vi "test_TCP_3_RT.vi"() -> ()   [LabVIEW 2014]
panel:
  out "error out":errorcluster
  in  "stop":bool
  out "string":string
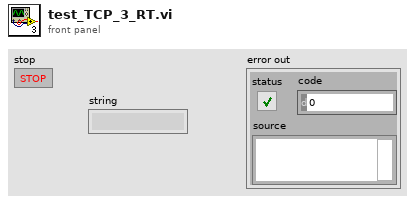
[diagram p1: front panel]
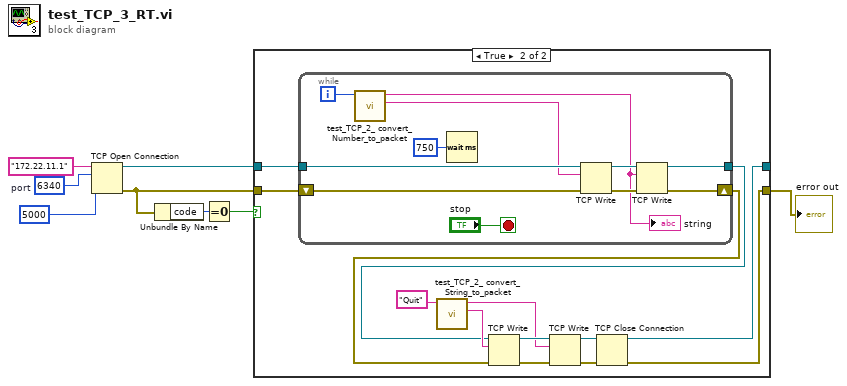
[diagram p0: block diagram]
diagram:
  w8 = u16 6340  # port
  n1 = TCP Open Connection(address="172.22.11.1", remote port or service name=w8, timeout ms (60000)=5000) -> (connection ID=w3:refnum<k5>, error out=w2:errorcluster)  [unwired: 2 in]
  n2 = Unbundle By Name(w2) -> ("code"=w5:i32)
  n3 = Equal To 0?(x=w5) -> (x = 0?=w4:bool)
  n4 = case shown="True" w4 {
    tunnel: w3 -> [w10 w23]
    tunnel: w2 -> [w9 w22]
    tunnel: [w10 w12] -> _
    tunnel: [w9 w11] -> w1
    frame False {
    }
    frame True {
      n5 = while {
        tunnel: w23 -> [w29]
        shift-right: [w33] -> w14
        shift-left: w22 -> [w30]
        tunnel: [w32] -> w13
        i -> [w26]
        stop <- "stop" stop-if-true
        n6 = call "test_TCP_2_ convert_Number_to_packet.vi"("input_Number"=w26) -> ("output_PrePacket"=w24:string, "output_packet"=w25:string)  [unwired: 9 in]
        "string" <- w25
        n7 = Wait (ms)(milliseconds to wait=u32 750) -> ()  [unwired: 1 out]
        n8 = TCP Write(connection ID=w29, data in=w24, error in (no error)=w30) -> (connection ID out=w27:refnum<k5>, error out=w28:errorcluster)  [unwired: 1 in, 1 out]
        n9 = TCP Write(connection ID=w27, data in=w25, error in (no error)=w28) -> (connection ID out=w32:refnum<k5>, error out=w33:errorcluster)  [unwired: 2 out]
      }
      n10 = call "test_TCP_2_ convert_String_to_packet.vi"("input_string"="Quit" ("data in")) -> ("output_PrePacket"=w21:string, "output_packet"=w18:string)  [unwired: 9 in]
      n11 = TCP Write(connection ID=w13, data in=w21, error in (no error)=w14) -> (connection ID out=w20:refnum<k5>, error out=w19:errorcluster)  [unwired: 2 out]
      n12 = TCP Write(connection ID=w20, data in=w18, error in (no error)=w19) -> (connection ID out=w16:refnum<k5>, error out=w15:errorcluster)  [unwired: 2 out]
      n13 = TCP Close Connection(connection ID=w16, error in (no error)=w15) -> (connection ID out=w12:refnum<k5>, error out=w11:errorcluster)  [unwired: 1 in]
    }
  }
  "error out" <- w1
